vi "Periodic Tasks.vi"(7 "Chassis X SPD":dbl=0.65, 8 "error in":errorcluster) -> ()   [LabVIEW 2019]
doc: "This VI runs in parallel to other tasks. It can contain as many user-defined periodic loops as you need. These can carry out PID or other sorts of timed response."
uses:
  <vilib>/Rock Robotics/WPI/Utilities/WPI_GetSetVariantRefNum.vi
  Robot Global Data.vi
  <vilib>/Rock Robotics/Network Tables/NT Write Boolean.vi
  <vilib>/Rock Robotics/Network Tables/NT Read Number.vi
  <vilib>/Rock Robotics/Network Tables/NT Write Number.vi
  <vilib>/Rock Robotics/WPI/RobotDrive/WPI_RobotDriveArcadeDrive_Standard(NoSaturation).vi
  <vilib>/Analysis/NI_AALPro.lvlib
panel:
  in  "Chassis Y SPD":dbl=0.65
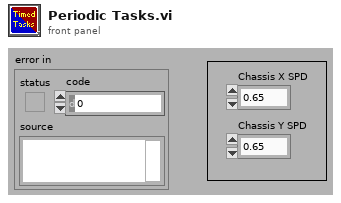
[diagram p1: front panel]
types:
  T1 = typedef "WPI_MotorControlDeviceRef.ctl" = cluster{"DeviceStatus":errorcluster, "Type":T2, "PWM":cluster{"PWM Channel":T3, "DeadBand":T4}, "CAN":cluster{"Device Number":u8, "SetOutput VI Ref":variant, "GetOutput VI Ref":variant, "Enable VI Ref":variant, "Disable VI Ref":variant, "Data":variant}, "Invert":bool, "DIO PWM":cluster{"PWM \"Enable\" Channel":T3, "DIOChannel":T5, "PWM Rate":dbl}}
  T2 = typedef "WPI_MotorControlType.ctl" = enum16{"PWM", "CAN", "DIO PWM"}
  T3 = typedef "FPGA_DIOPWMChannel.ctl" = enum8{"PWM 0", "PWM 1", "PWM 2", "PWM 3", "PWM 4", "PWM 5", "PWM 6", "PWM 7", "PWM 8", "PWM 9", "PWM MXP 0", "PWM MXP 1", "PWM MXP 2", "PWM MXP 3", "PWM MXP 4", "PWM MXP 5", "PWM MXP 6", "PWM MXP 7", "PWM MXP 8", "PWM MXP 9", "Invalid"}
  T4 = typedef "WPI_PWMDeadband.ctl" = cluster{"Name":string, "maxPositivePwm":i32, "minPositivePwm":i32, "centerPwm":i32, "maxNegativePwm":i32, "minNegativePwm":i32, "angularRange":u16}
  T5 = typedef "FPGA_DIOChannel.ctl" = enum8{"DIO 0", "DIO 1", "DIO 2", "DIO 3", "DIO 4", "DIO 5", "DIO 6", "DIO 7", "DIO 8", "DIO 9", "DIO MXP 0", "DIO MXP 1", "DIO MXP 2", "DIO MXP 3", "DIO MXP 4", "DIO MXP 5", "DIO MXP 6", "DIO MXP 7", "DIO MXP 8", "DIO MXP 9", "DIO MXP 10", "DIO MXP 11", "DIO MXP 12", "DIO MXP 13", "DIO MXP 14", "DIO MXP 15", "SPI Port CS1", "SPI Port CS2", "SPI Port CS3", "SPI Port MISO", "SPI Port MOSI", "Invalid"}
  T6 = typedef "WPI_JoystickDevRef.ctl" = cluster{"Device":T7}
  T7 = typedef "WPI_JoystickDeviceEnum.ctl" = enum16{"USB 0", "USB 1", "USB 2", "USB 3", "USB 4", "USB 5"}
  T8 = typedef "WPI_RobotDriveDevRef.ctl" = cluster{"DevStatus":errorcluster, "Motors[]":T1[], "Square Inputs":bool, "Max Output":dbl}
  T9 = cluster{"JoystickDevRef":T6, "RobotDriveDevRef":T8}
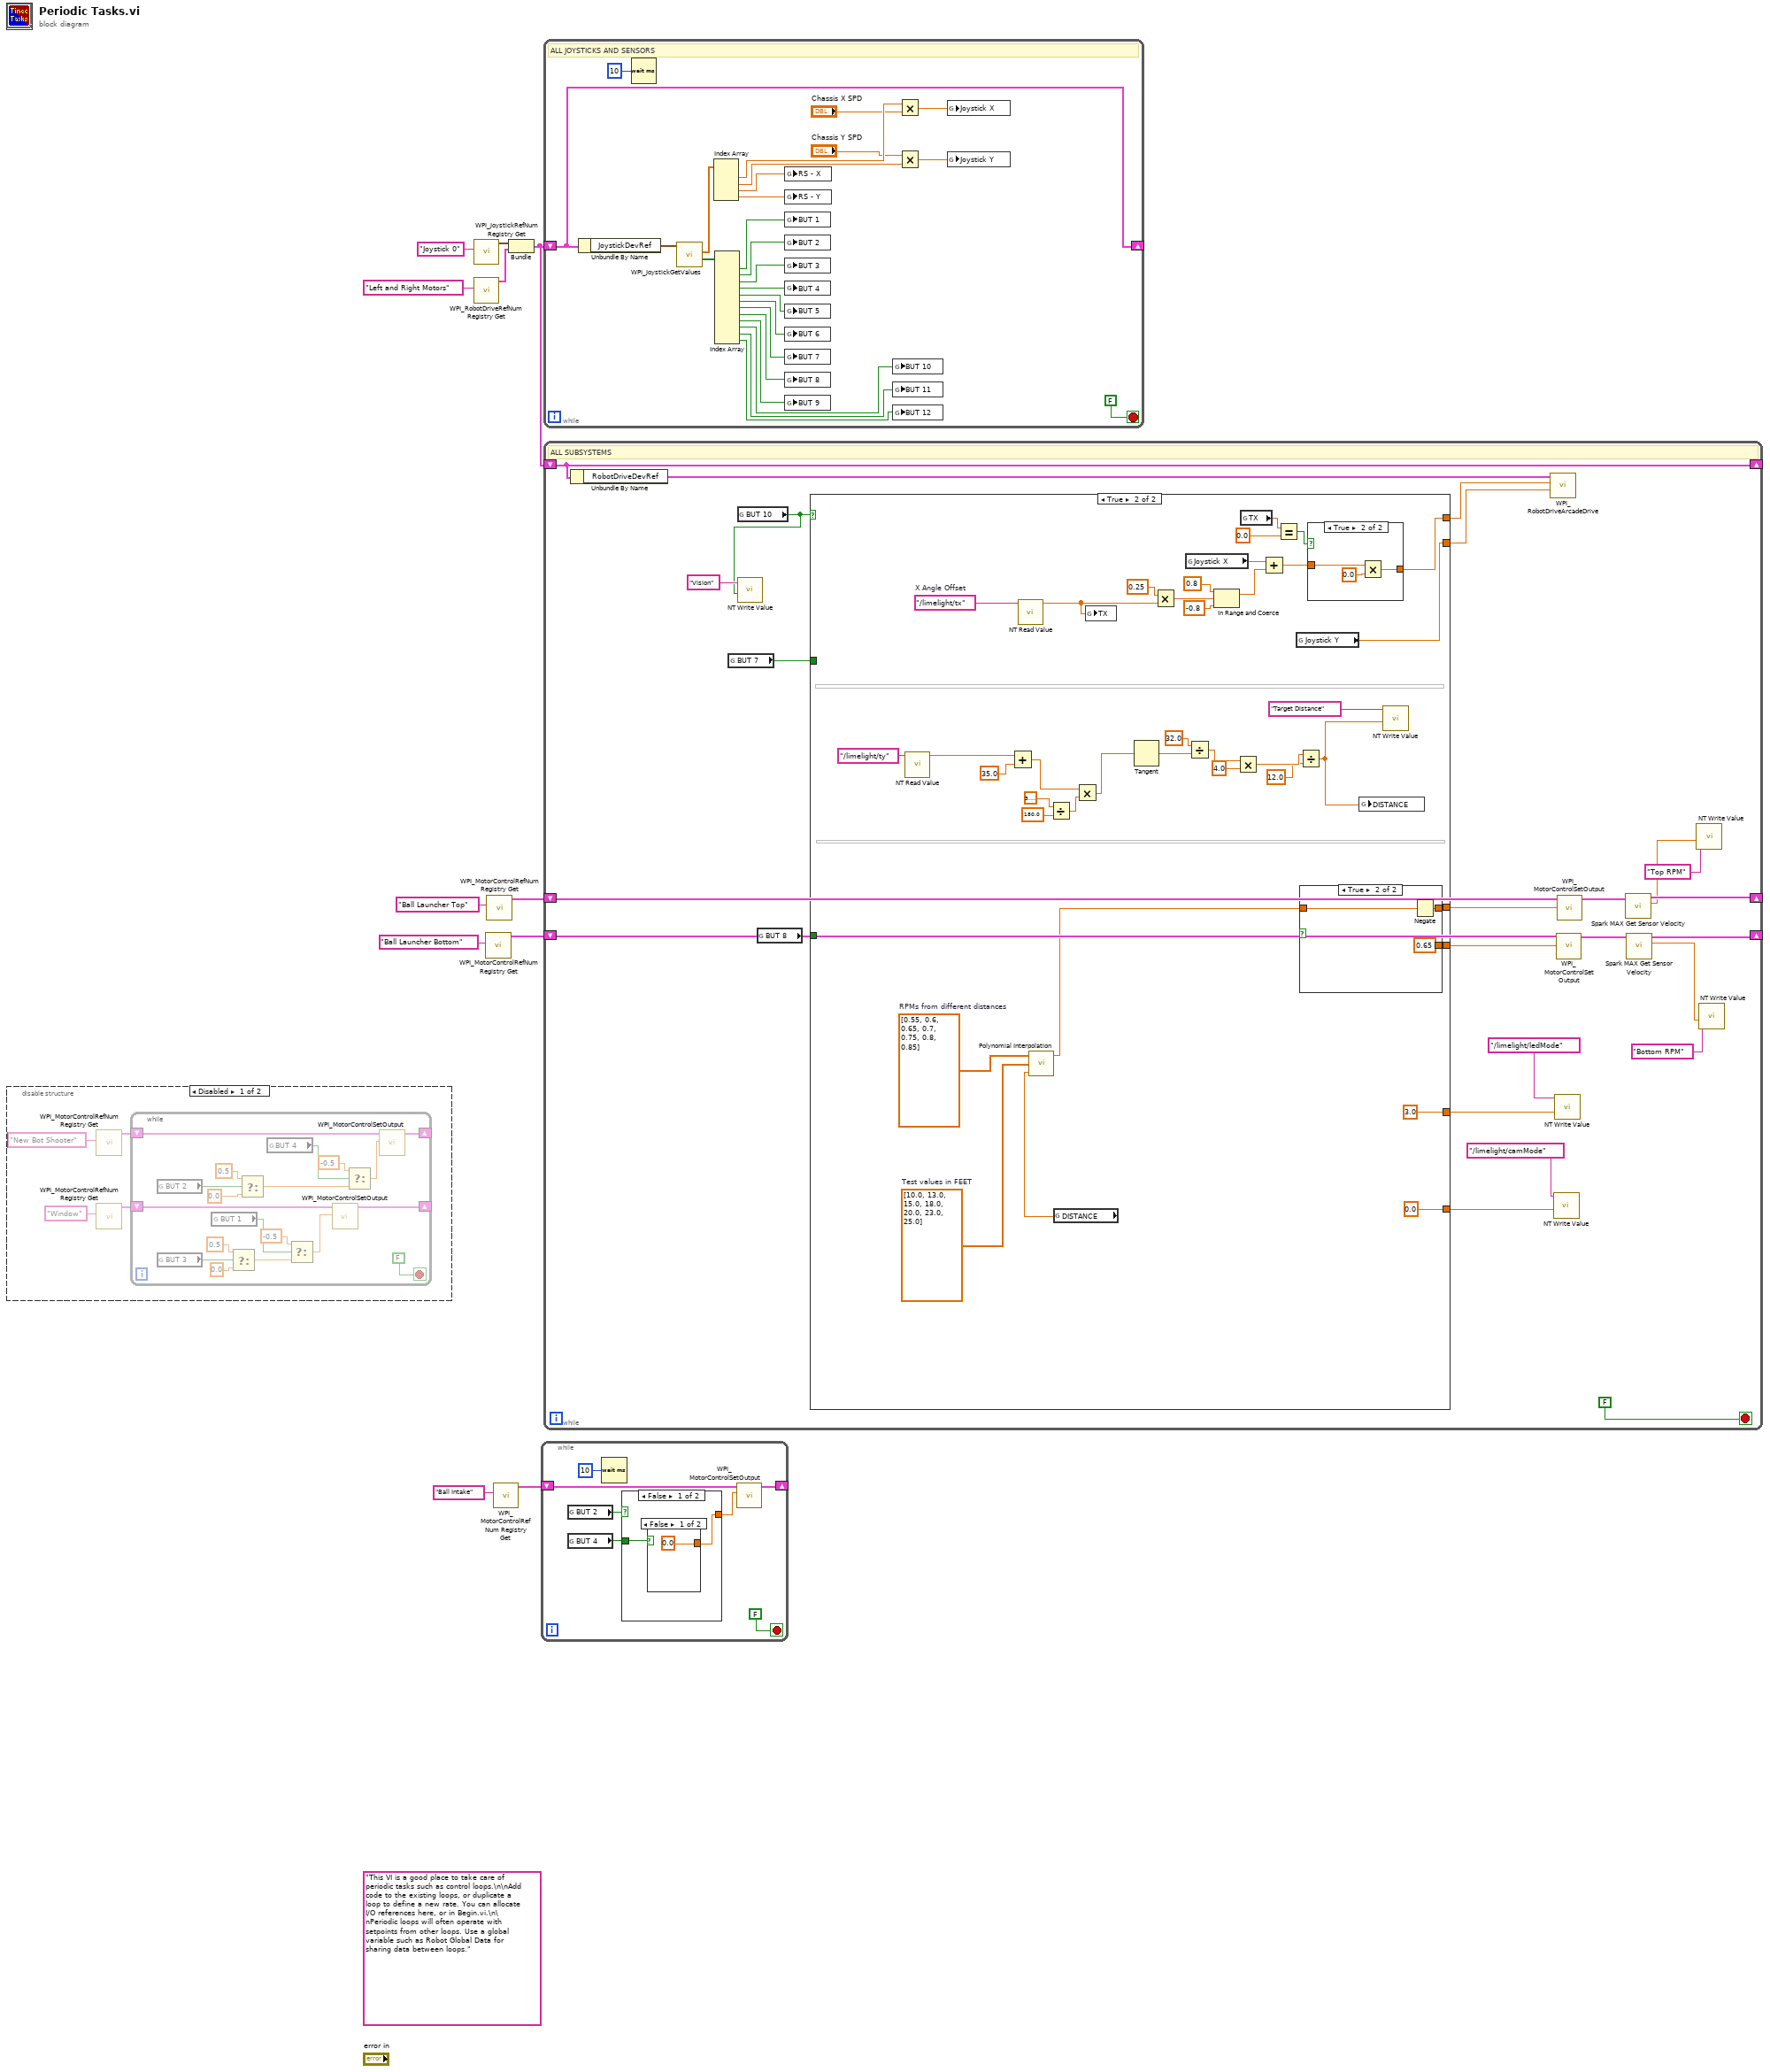
[diagram p0: block diagram]
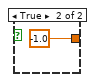
[diagram p3: hidden frame]
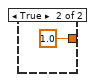
[diagram p4: hidden frame]
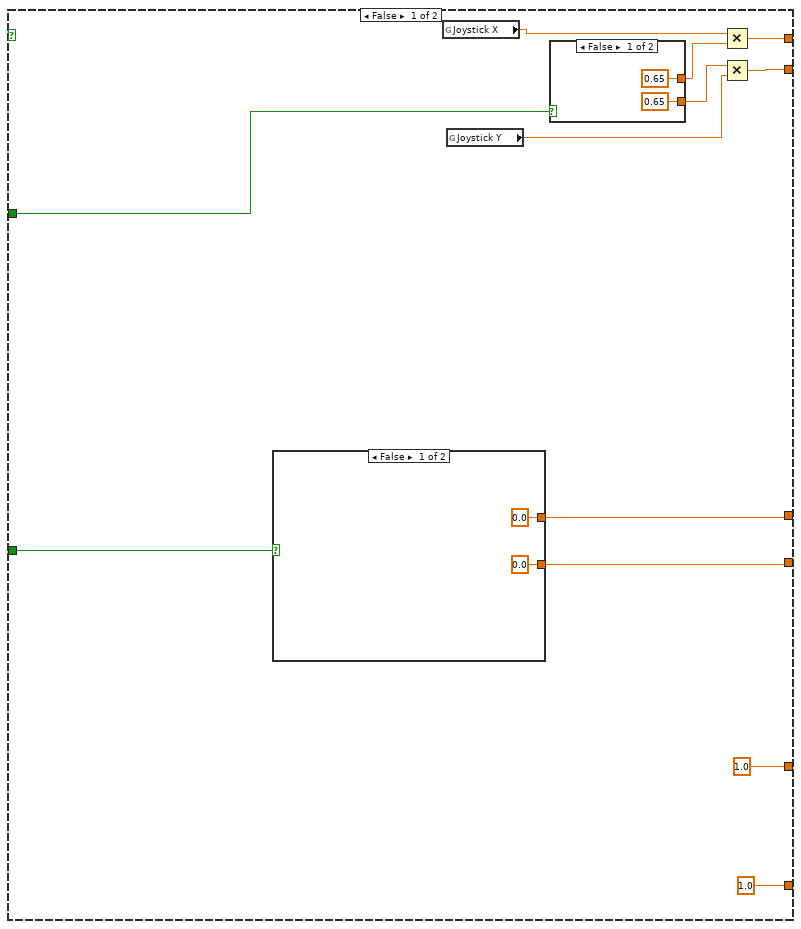
[diagram p5: hidden frame]
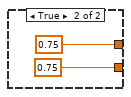
[diagram p6: hidden frame]
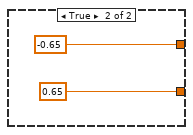
[diagram p7: hidden frame]
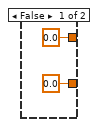
[diagram p8: hidden frame]
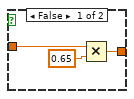
[diagram p9: hidden frame]
diagram:
  (unwired) "This VI is a good place to take care of periodic tasks such as control loops.\n\nAdd code to the existing loops, or duplicate a loop to define a new rate. You can allocate I/O references here, or in Begin.vi.\n\nPeriodic loops will often operate with setpoints from other loops. Use a global variable such as Robot Global Data for sharing data between loops."
  n1 = disable-structure shown="Disabled" {
    frame Disabled {
      n2 = call <vilib>:"WPI_MotorControlRefNum Registry Get.vi"("refnum name"="New Bot Shooter") -> ("MotorControlDevRef"=w12:T1)  [unwired: 9 in, 1 out]
      n3 = call <vilib>:"WPI_MotorControlRefNum Registry Get.vi"("refnum name"="Window") -> ("MotorControlDevRef"=w15:T1)  [unwired: 9 in, 1 out]
      n4 = while {
        shift-right: [w33] -> _
        shift-left: w15 -> [w32]
        shift-right: [w24] -> _
        shift-left: w12 -> [w23]
        stop <- FALSE stop-if-true
        n5 = global read "Robot Global Data.vi" "BUT 2"() -> (w18:bool)
        n6 = global read "Robot Global Data.vi" "BUT 3"() -> (w31:bool)
        n7 = global read "Robot Global Data.vi" "BUT 1"() -> (w27:bool)
        n8 = Select(t=0.5, s=w31, f=0.0) -> (s? t:f=w28:dbl)
        n9 = Select(t=0.5, s=w18, f=0.0) -> (s? t:f=w21:dbl)
        n10 = global read "Robot Global Data.vi" "BUT 4"() -> (w22:bool)
        n11 = Select(t=-0.5, s=w27, f=w28) -> (s? t:f=w25:dbl)
        n12 = call <vilib>:"WPI_MotorControlSetOutput.vi"("Output"=w25, "MotorControlDevRef"=w32) -> ("MotorControlDevRef"=w33:T1)  [unwired: 7 in, 2 out]
        n13 = Select(t=-0.5, s=w22, f=w21) -> (s? t:f=w17:dbl)
        n14 = call <vilib>:"WPI_MotorControlSetOutput.vi"("Output"=w17, "MotorControlDevRef"=w23) -> ("MotorControlDevRef"=w24:T1)  [unwired: 7 in, 2 out]
      }
    }
    frame Enabled {
    }
  }
  n15 = call <vilib>:"WPI_JoystickRefNum Registry Get.vi"("refnum name"="Joystick 0") -> ("JoystickDevRef"=w9:T6)  [unwired: 1 in, 9 out]
  n16 = call <vilib>:"WPI_RobotDriveRefNum Registry Get.vi"("refnum name"="Left and Right Motors") -> ("RobotDriveDevRef"=w8:T8)  [unwired: 1 in, 9 out]
  n17 = call <vilib>:"WPI_MotorControlRefNum Registry Get.vi"("refnum name"="Ball Launcher Bottom") -> ("MotorControlDevRef"=w1:T1)  [unwired: 9 in, 1 out]
  n18 = call <vilib>:"WPI_MotorControlRefNum Registry Get.vi"("refnum name"="Ball Launcher Top") -> ("MotorControlDevRef"=w4:T1)  [unwired: 9 in, 1 out]
  n19 = call <vilib>:"WPI_MotorControlRefNum Registry Get.vi"("refnum name"="Ball Intake") -> ("MotorControlDevRef"=w6:T1)  [unwired: 9 in, 1 out]
  n20 = Bundle("JoystickDevRef"=w9, "RobotDriveDevRef"=w8) -> (w7:T9)  [unwired: 1 out]
  n21 = while {
    shift-right: [w38] -> _
    shift-left: w6 -> [w37]
    stop <- FALSE stop-if-true
    n22 = global read "Robot Global Data.vi" "BUT 2"() -> (w40:bool)
    n23 = global read "Robot Global Data.vi" "BUT 4"() -> (w41:bool)
    n24 = Wait (ms)(milliseconds to wait=u32 10) -> ()  [unwired: 1 out]
    n25 = case shown="False" w40 {
      tunnel: [w43 1.0 ("Output")] -> w39
      tunnel: w41 -> [w42 _]
      frame False {
        n26 = case shown="False" w42 {
          tunnel: [0.0 ("Output") -1.0 ("Output")] -> w43
          frame False {
          }
          frame True {
          }
        }
      }
      frame True {
      }
    }
    n27 = call <vilib>:"WPI_MotorControlSetOutput.vi"("Output"=w39, "MotorControlDevRef"=w37) -> ("MotorControlDevRef"=w38:T1)  [unwired: 7 in, 2 out]
  }
  n28 = while {
    shift-right: [w56] -> _
    shift-left: w7 -> [w56]
    stop <- FALSE stop-if-true
    # "ALL JOYSTICKS AND SENSORS"
    n29 = Unbundle By Name(w56) -> ("JoystickDevRef"=w70:T6)
    n30 = Wait (ms)(milliseconds to wait=u32 10) -> ()  [unwired: 1 out]
    n31 = call <vilib>:"WPI_JoystickGetValues.vi"("JoystickDevRef"=w70) -> ("Buttons"=w69:bool[], "Axes"=w55:dbl[])  [unwired: 6 in, 3 out]
    n32 = Index Array(array=w55) -> (element #1=w52:dbl, element #2=w51:dbl, element #3=w48:dbl, element #4=w47:dbl)  [unwired: 4 in]
    n33 = Index Array(array=w69) -> (element #1=w68:bool, element #2=w67:bool, element #3=w66:bool, element #4=w65:bool, element #5=w64:bool, element #6=w63:bool, element #7=w62:bool, element #8=w61:bool, element #9=w60:bool, element #10=w59:bool, element #11=w58:bool, element #12=w57:bool)  [unwired: 12 in]
    n34 = global write "Robot Global Data.vi" "RS - X"(w48) -> ()
    n35 = global write "Robot Global Data.vi" "RS - Y"(w47) -> ()
    n36 = global write "Robot Global Data.vi" "BUT 1"(w68) -> ()
    n37 = global write "Robot Global Data.vi" "BUT 2"(w67) -> ()
    n38 = global write "Robot Global Data.vi" "BUT 3"(w66) -> ()
    n39 = global write "Robot Global Data.vi" "BUT 4"(w65) -> ()
    n40 = global write "Robot Global Data.vi" "BUT 5"(w64) -> ()
    n41 = global write "Robot Global Data.vi" "BUT 6"(w63) -> ()
    n42 = global write "Robot Global Data.vi" "BUT 7"(w62) -> ()
    n43 = global write "Robot Global Data.vi" "BUT 8"(w61) -> ()
    n44 = global write "Robot Global Data.vi" "BUT 9"(w60) -> ()
    n45 = global write "Robot Global Data.vi" "BUT 10"(w59) -> ()
    n46 = global write "Robot Global Data.vi" "BUT 11"(w58) -> ()
    n47 = global write "Robot Global Data.vi" "BUT 12"(w57) -> ()
    n48 = Multiply(x=w52, y="Chassis X SPD") -> (x*y=w54:dbl)
    n49 = Multiply(x="Chassis Y SPD", y=w51) -> (x*y=w53:dbl)
    n50 = global write "Robot Global Data.vi" "Joystick X"(w54) -> ()
    n51 = global write "Robot Global Data.vi" "Joystick Y"(w53) -> ()
  }
  n52 = while {
    shift-right: [w96] -> _
    shift-left: w7 -> [w96]
    shift-right: [w78] -> _
    shift-left: w4 -> [w86]
    shift-right: [w80] -> _
    shift-left: w1 -> [w85]
    stop <- FALSE stop-if-true
    # "ALL SUBSYSTEMS"
    n53 = Unbundle By Name(w96) -> ("RobotDriveDevRef"=w95:T8)
    n54 = global read "Robot Global Data.vi" "BUT 7"() -> (w73:bool)
    n55 = global read "Robot Global Data.vi" "BUT 10"() -> (w87:bool)
    n56 = call-poly <vilib>:"NT Write Value.vi"("Boolean"=w87, "Name"="Vision") -> ()  [unwired: 9 in, 1 out]
    n57 = global read "Robot Global Data.vi" "BUT 8"() -> (w82:bool)
    n58 = case shown="True" w87 {
      tunnel: [w104 w148] -> w94
      tunnel: [w103 w144] -> w93
      tunnel: [1.0 ("Numeric") 0.0 ("Numeric")] -> w90
      tunnel: [1.0 ("Numeric") 3.0 ("Numeric")] -> w89
      tunnel: [w107 w121] -> w84
      tunnel: [w106 w119] -> w83
      tunnel: w82 -> [w105 w118]
      tunnel: w73 -> [w98 _]
      frame False {
        n59 = case shown="False" w105 {
          tunnel: [0.0 ("Output") -0.65 ("Output")] -> w107
          tunnel: [0.0 ("Output") 0.65 ("Output")] -> w106
          frame False {
          }
          frame True {
          }
        }
        n60 = global read "Robot Global Data.vi" "Joystick X"() -> (w101:dbl)
        n61 = global read "Robot Global Data.vi" "Joystick Y"() -> (w102:dbl)
        n62 = case shown="False" w98 {
          tunnel: [0.65 ("x") 0.75 ("x")] -> w100
          tunnel: [0.65 ("y") 0.75 ("y")] -> w99
          frame False {
          }
          frame True {
          }
        }
        n63 = Multiply(x=w101, y=w99) -> (x*y=w104:dbl)
        n64 = Multiply(x=w100, y=w102) -> (x*y=w103:dbl)
      }
      frame True {
        w124 = dbl[] [10.0, 13.0, 15.0, 18.0, 20.0, 23.0, 25.0]  # Test values in FEET
        w125 = dbl[] [0.55, 0.6, 0.65, 0.7, 0.75, 0.8, 0.85]  # RPMs from different distances
        w156 = "/limelight/tx"  # X Angle Offset
        n65 = call-poly <vilib>:"NT Read Value.vi"("Name"="/limelight/ty") -> ("Numeric"=w135:dbl)  [unwired: 9 in, 1 out]
        n66 = Add(x=w135, y=35.0) -> (x+y=w133:dbl)
        n67 = call-poly <vilib>:"NT Read Value.vi"("Name"=w156) -> ("Numeric"=w143:dbl)  [unwired: 9 in, 1 out]
        n68 = Divide(x=3.141592653589793, y=180.0) -> (x/y=w136:dbl)
        n69 = global read "Robot Global Data.vi" "DISTANCE"() -> (w122:dbl)
        n70 = call <vilib>:"Polynomial Interpolation.vi"("x value"=w122, "X"=w124, "Y"=w125) -> ("interpolation value"=w120:dbl)  [unwired: 2 out]
        n71 = Multiply(x=w133, y=w136) -> (x*y=w132:dbl)
        n72 = global write "Robot Global Data.vi" "TX"(w143) -> ()
        n73 = Tangent(1:w132) -> (0:w142:dbl)
        n74 = Multiply(x=0.25 ("y"), y=w143) -> (x*y=w153:dbl)
        n75 = global read "Robot Global Data.vi" "Joystick X"() -> (w155:dbl)
        n76 = Divide(x=32.0, y=w142) -> (x/y=w131:dbl)
        n77 = In Range and Coerce(upper limit=0.8, x=w153, lower limit=-0.8) -> (coerced(x)=w154:dbl)  [unwired: 1 out]
        n78 = Multiply(x=w131, y=4.0) -> (x*y=w129:dbl)
        n79 = global read "Robot Global Data.vi" "TX"() -> (w146:dbl)
        n80 = Add(x=w155, y=w154) -> (x+y=w149:dbl)
        n81 = Equal?(x=w146, y=0.0) -> (x = y?=w147:bool)
        n82 = global read "Robot Global Data.vi" "Joystick Y"() -> (w144:dbl)
        n83 = Divide(x=w129, y=12.0) -> (x/y=w123:dbl)
        n84 = case shown="True" w118 {
          tunnel: [0.0 w161] -> w121
          tunnel: w120 -> [_ w160]
          tunnel: [0.0 ("Output") 0.65 ("Output")] -> w119
          frame False {
          }
          frame True {
            n85 = Negate(x=w160) -> (-x=w161:dbl)
          }
        }
        n86 = case shown="True" w147 {
          tunnel: w149 -> [w163 w167]
          tunnel: [w164 w165] -> w148
          frame False {
            n87 = Multiply(x=w163, y=0.65) -> (x*y=w164:dbl)
          }
          frame True {
            n88 = Multiply(x=w167, y=0.0) -> (x*y=w165:dbl)
          }
        }
        n89 = global write "Robot Global Data.vi" "DISTANCE"(w123) -> ()
        n90 = call-poly <vilib>:"NT Write Value.vi"("Numeric"=w123, "Name"="Target Distance") -> ()  [unwired: 9 in, 1 out]
      }
    }
    n91 = call-poly <vilib>:"WPI_RobotDriveArcadeDrive.vi"("Y axis value"=w93, "X axis value"=w94, "RobotDriveDevRef"=w95) -> ()  [unwired: 6 in, 3 out]
    n92 = call-poly <vilib>:"NT Write Value.vi"("Numeric"=w90, "Name"="/limelight/camMode") -> ()  [unwired: 9 in, 1 out]
    n93 = call-poly <vilib>:"NT Write Value.vi"("Numeric"=w89, "Name"="/limelight/ledMode") -> ()  [unwired: 9 in, 1 out]
    n94 = call <vilib>:"WPI_MotorControlSetOutput.vi"("Output"=w83, "MotorControlDevRef"=w85) -> ("MotorControlDevRef"=w81:T1)  [unwired: 7 in, 2 out]
    n95 = call <vilib>:"WPI_MotorControlSetOutput.vi"("Output"=w84, "MotorControlDevRef"=w86) -> ("MotorControlDevRef"=w79:T1)  [unwired: 7 in, 2 out]
    n96 = call <vilib>:"Spark MAX Get Sensor Velocity.vi"("MotorControlDevRef in"=w79) -> ("Sensor Velocity"=w75:dbl, "MotorControlDevRef out"=w78:T1)  [unwired: 7 in, 2 out]
    n97 = call <vilib>:"Spark MAX Get Sensor Velocity.vi"("MotorControlDevRef in"=w81) -> ("Sensor Velocity"=w77:dbl, "MotorControlDevRef out"=w80:T1)  [unwired: 7 in, 2 out]
    n98 = call-poly <vilib>:"NT Write Value.vi"("Numeric"=w75, "Name"="Top RPM") -> ()  [unwired: 9 in, 1 out]
    n99 = call-poly <vilib>:"NT Write Value.vi"("Numeric"=w77, "Name"="Bottom RPM") -> ()  [unwired: 9 in, 1 out]
  }
